vi "Filter Meta.vi"(8 "error in (no error)":errorcluster, 10 "Element":refnum<class "Config Element.lvclass">, 11 "Config Storage in":refnum<class "Config Storage.lvclass">) -> (0 "error out":errorcluster, 2 "Filtered Meta":T1[](array[typedef]), 3 "Config Storage out":refnum<class "Config Storage.lvclass">)   [LabVIEW 2020, in "CDM-Config.lvlib" / "Config Storage.lvclass"]
uses:
  Config Storage.lvclass
  Config Element/Config Element.lvclass
  Meta Data.ctl
  CDM-Config.lvlib
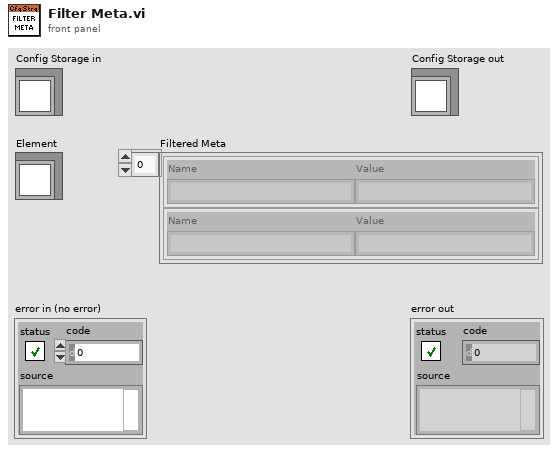
[diagram p1: front panel]
types:
  T1 = typedef "CDM-Config.lvlib/Meta Data.ctl" = cluster{"Name":string, "Value":string}
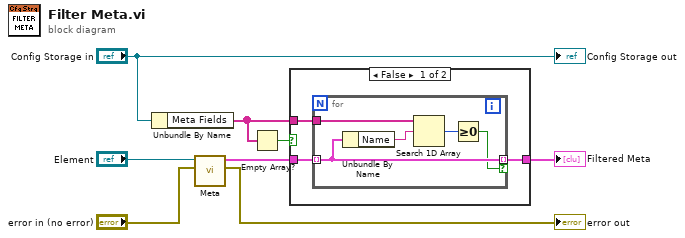
[diagram p0: block diagram]
diagram:
  n1 = Unbundle By Name("Config Storage in") -> ("Meta Fields"=w6:string[])
  n2 = call "Meta.vi"("error in (no error)"="error in (no error)", "Config Element in"="Element") -> ("error out"=→"error out":errorcluster, "Meta Data"=w8:T1[])  [unwired: 8 in]
  n3 = Empty Array?(array=w6) -> (empty?=w5:bool)
  n4 = case shown="False" w5 {
    tunnel: w8 -> [w11 w17]
    tunnel: [w10 w17] -> w7
    tunnel: w6 -> [w9 _]
    frame False {
      n5 = for {
        tunnel: w9 -> [w16]
        tunnel: w11 -> [w15] mode=indexing
        tunnel: [w15] -> w10 mode=indexing if=w12
        n6 = Unbundle By Name(w15) -> ("Name"=w14:string)
        n7 = Search 1D Array(1D array=w16, element=w14) -> (index of element=w13:i32)  [unwired: 1 in]
        n8 = Greater Or Equal To 0?(x=w13) -> (x >= 0?=w12:bool)
      }
    }
    frame True {
    }
  }
  "Filtered Meta" <- w7
  "Config Storage out" <- "Config Storage in"
